vi "New Bundle Definition.vi"(8 "error in (no error)":errorcluster, 11 "Bundle Builder in":refnum<class "Bundle Builder.lvclass">) -> (0 "error out":errorcluster, 2 "Cancelled?":bool, 3 "Bundle Builder out":refnum<class "Bundle Builder.lvclass">, 4 "Bundle Filename":string)   [LabVIEW 2020, in "Bundle Builder.lvclass"]
uses:
  Bundle Builder.lvclass
  Bundle Builder.lvclass/Bundle Builder.ctl
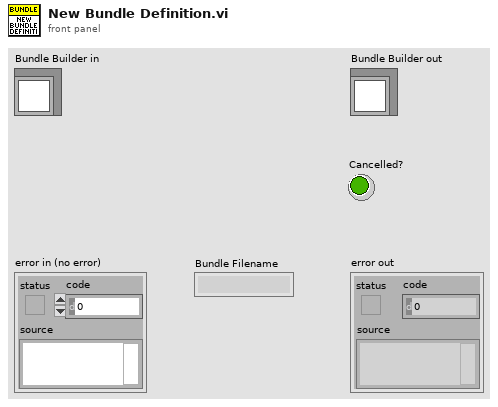
[diagram p1: front panel]
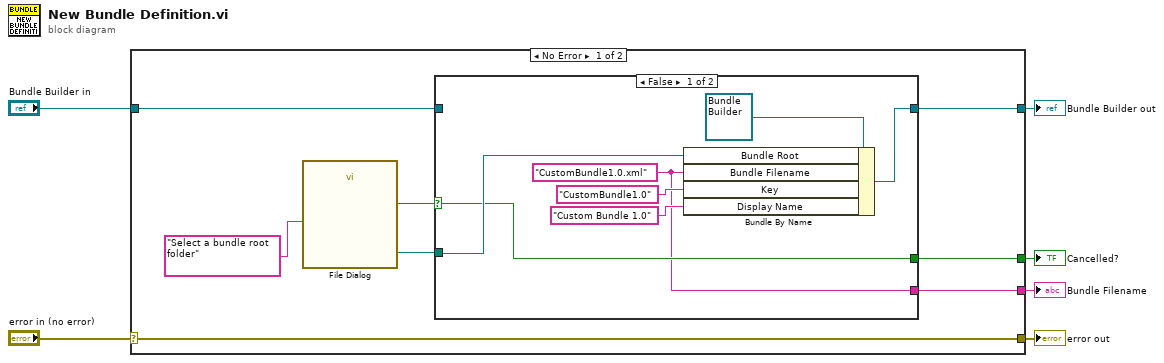
[diagram p0: block diagram]
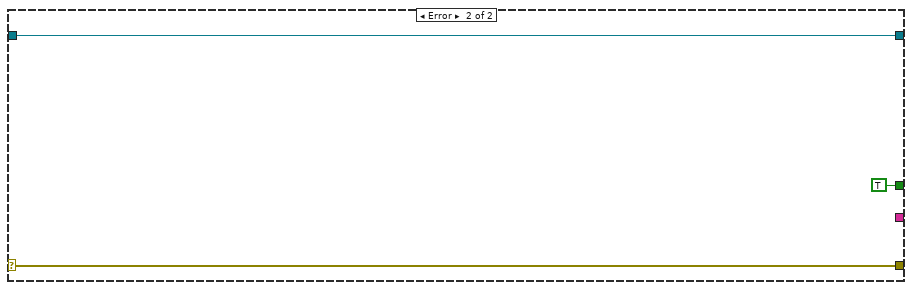
[diagram p3: hidden frame]
diagram:
  n1 = case shown="No Error" "error in (no error)" {
    selector: "error in (no error)" -> [w9 w26]
    tunnel: [w9 w26] -> w5
    tunnel: [w10 w25] -> w3
    tunnel: "Bundle Builder in" -> [w11 w25]
    tunnel: [w8 TRUE] -> w2
    tunnel: [w7 _] -> w1
    frame No Error {
      n2 = call "File Dialog"("prompt"="Select a bundle root folder") -> ("selected path"=w12:path, "cancelled"=w13:bool)  [unwired: 11 in, 2 out]
      n3 = case shown="False" w13 {
        selector: w13 -> [w16 w22]
        tunnel: w12 -> [w20 _]
        tunnel: w11 -> [_ w23]
        tunnel: [w17 w23] -> w10
        tunnel: [w16 w22] -> w8
        tunnel: [w15 _] -> w7
        frame False {
          w15 = "CustomBundle1.0.xml" ("Bundle Filename")
          n4 = Bundle By Name(cluster=refnum<class "Bundle Builder.lvclass"> refnum ("Bundle Builder in"), "Bundle Root"=w20, "Bundle Filename"=w15, "Key"="CustomBundle1.0" ("Bundle Filename"), "Display Name"="Custom Bundle 1.0" ("Bundle Filename")) -> (w17:refnum<class "Bundle Builder.lvclass">)
        }
        frame True {
        }
      }
    }
    frame Error {
    }
  }
  "error out" <- w5
  "Bundle Builder out" <- w3
  "Cancelled?" <- w2
  "Bundle Filename" <- w1
